vi "Magnet_rotation_control_V1.vi"() -> ()   [LabVIEW 2017]
uses:
  <vilib>/Instr/_visa.llb/VISA Configure Serial Port (Instr).vi
panel:
  in  "UPDATE CALIBRATION":bool
  in  "CALIBRATION ANGLE":dbl min=-10.0 max=370.0
  out "Error out":errorcluster
  out "String":string
  in  "Speed":dbl min=1.0 max=100.0
  in  "stop/start":bool
  in  "Target angle":dbl min=-10.0 max=370.0
  in  "clockwise/anticlockwise":bool
  in  "Stop":bool
  in  "COM Port":refnum<visa-resource-name>
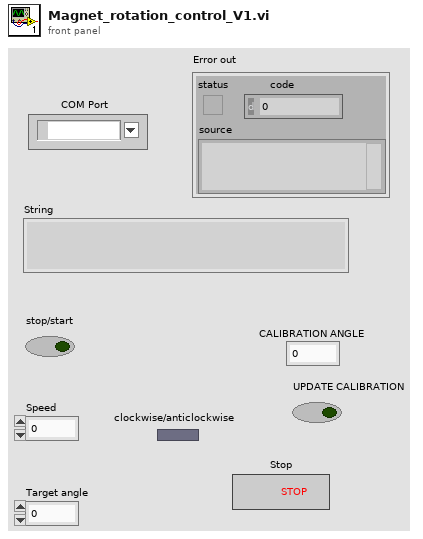
[diagram p1: front panel]
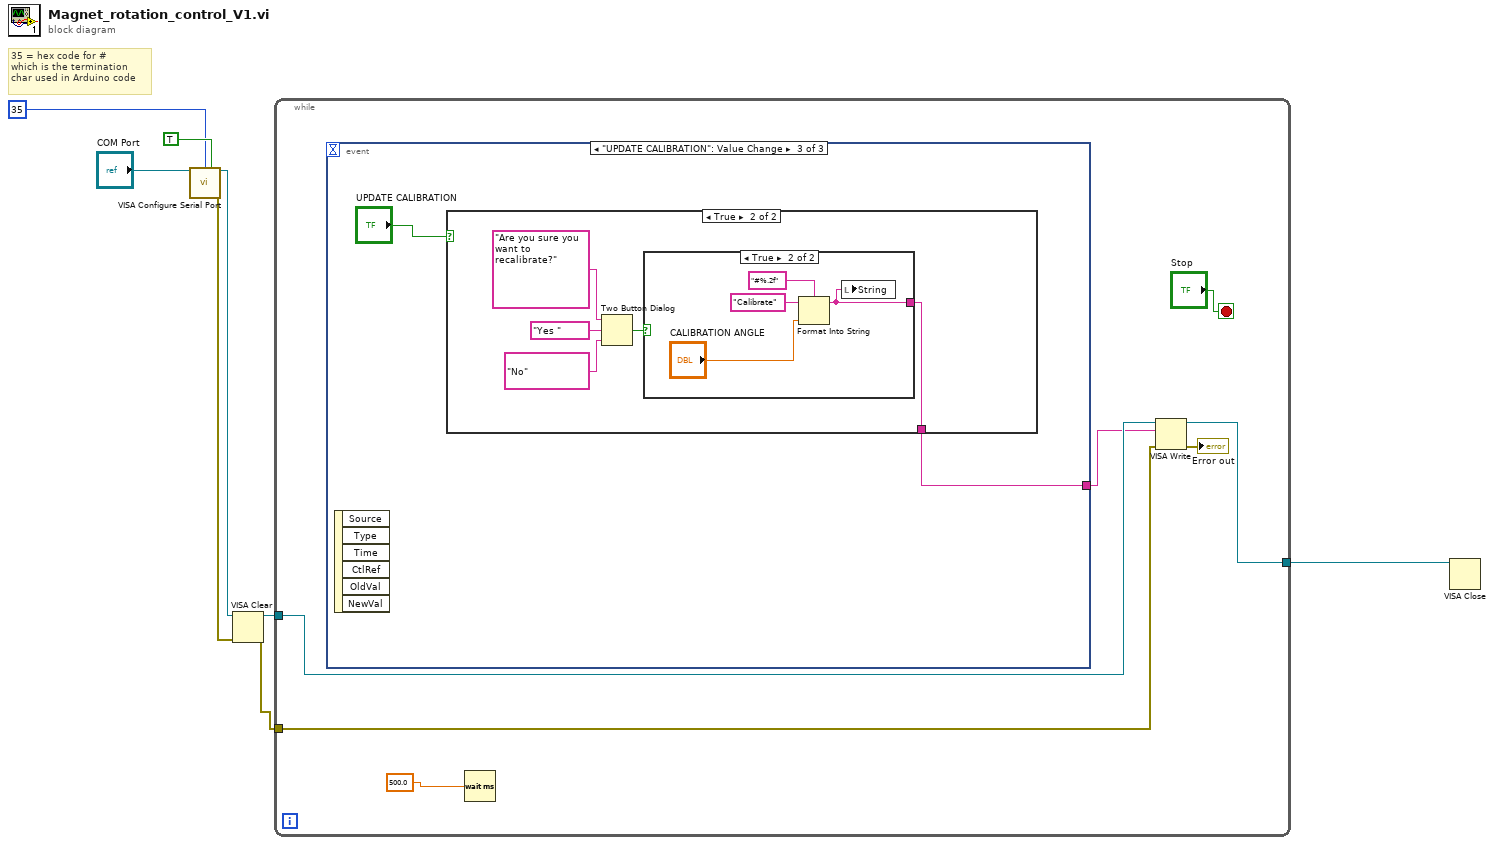
[diagram p0: block diagram]
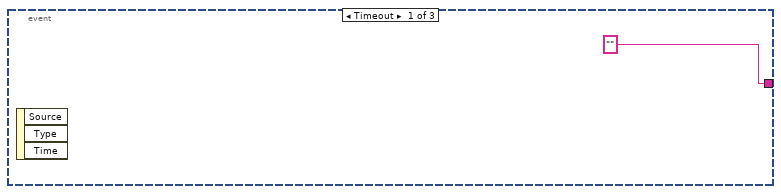
[diagram p2: hidden frame]
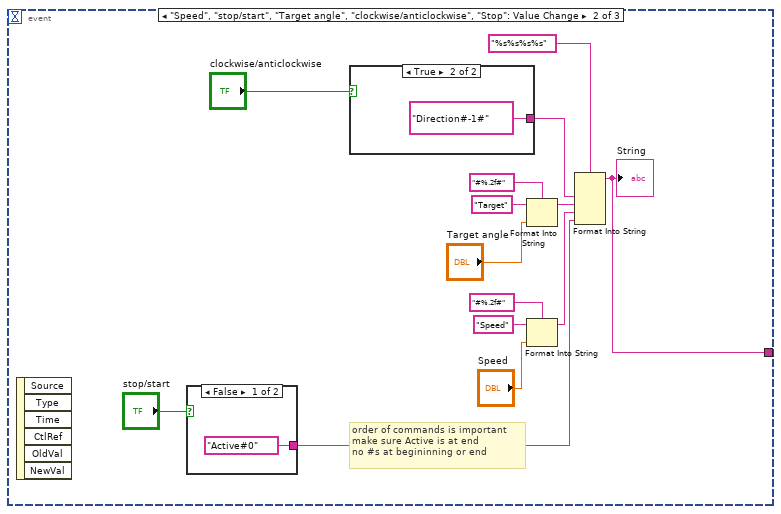
[diagram p3: hidden frame]
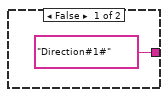
[diagram p4: hidden frame]
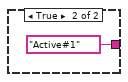
[diagram p5: hidden frame]
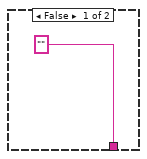
[diagram p6: hidden frame]
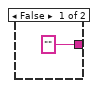
[diagram p7: hidden frame]
diagram:
  # "35 = hex code for #\nwhich is the termination \nchar used in Arduino code"
  n1 = call-poly "VISA Configure Serial Port"("VISA resource name"="COM Port", "termination char\n(0xA = '\\n' = LF)"=35, "Enable Termination\nChar (T)"=TRUE ("Enable Termination\nChar (T)")) -> ("VISA resource name out"=w4:refnum<visa-resource-name>, "error out"=w5:errorcluster)  [unwired: 11 in]
  n2 = VISA Clear(VISA resource name=w4, error in (no error)=w5) -> (VISA resource name out=w3:refnum<visa-resource-name>, error out=w2:errorcluster)
  n3 = while {
    tunnel: w3 -> [w14]
    tunnel: w2 -> [w13]
    tunnel: [w9] -> w1
    stop <- "Stop" stop-if-true
    n4 = event shown="[2] \"UPDATE CALIBRATION\": Value Change" {
      selector: _ -> [_ _ _]
      dyn-events: _ -> [_ _ _]
      timeout: _ -> [_ _ _]
      tunnel: ["" w21 w35] -> w12
      event Timeout {
        n5 = event-data() -> ()  [unwired: 1 in, 3 out]
      }
      event "Speed", "stop/start", "Target angle", "clockwise/anticlockwise", "Stop": Value Change {
        # "order of commands is important\nmake sure Active is at end\nno #s at begininning or end"
        n6 = event-data() -> ()  [unwired: 1 in, 6 out]
        n7 = case shown="False" "stop/start" {
          tunnel: ["Active#0" "Active#1"] -> w17
          frame False {
          }
          frame True {
          }
        }
        n8 = case shown="True" "clockwise/anticlockwise" {
          tunnel: ["Direction#1#" "Direction#-1#"] -> w20
          frame False {
          }
          frame True {
          }
        }
        n9 = Format Into String(format string="#%.2f#", initial string="Target" ("format string"), "Target angle") -> (resulting string=w19:string)  [unwired: 1 in, 1 out]
        n10 = Format Into String(format string="#%.2f#", initial string="Speed" ("format string"), "Speed") -> (resulting string=w18:string)  [unwired: 1 in, 1 out]
        n11 = Format Into String(format string="%s%s%s%s", w20, w19, w18, w17) -> (resulting string=w21:string)  [unwired: 2 in, 1 out]
        "String" <- w21
      }
      event "UPDATE CALIBRATION": Value Change {
        n12 = event-data() -> ()  [unwired: 1 in, 6 out]
        n13 = case shown="True" "UPDATE CALIBRATION" {
          tunnel: ["" w38] -> w35
          frame False {
          }
          frame True {
            n14 = Two Button Dialog(message="Are you sure you want to recalibrate?", 1:"No", 2:"Yes ") -> (T button?=w39:bool)
            n15 = case shown="True" w39 {
              tunnel: ["" w44] -> w38
              frame False {
              }
              frame True {
                n16 = Format Into String(format string="#%.2f", initial string="Calibrate" ("format string"), "CALIBRATION ANGLE") -> (resulting string=w44:string)  [unwired: 1 in, 1 out]
                n17 = local write "String"(w44) -> ()
              }
            }
          }
        }
      }
    }
    n18 = Wait (ms)(milliseconds to wait=500.0) -> ()  [unwired: 1 out]
    n19 = VISA Write(VISA resource name=w14, write buffer=w12, error in (no error)=w13) -> (VISA resource name out=w9:refnum<visa-resource-name>, error out=→"Error out":errorcluster)  [unwired: 1 out]
  }
  n20 = VISA Close(VISA resource name=w1) -> ()  [unwired: 1 in, 1 out]
